vi "Update Connect Panel Doc.vi"(8 "error in (no error)":errorcluster, 11 "vi path":path) -> (0 "error out":errorcluster, 3 "Array":T1(array[cluster]))   [LabVIEW 2017]
uses:
  Communicable State Machine.lvlib
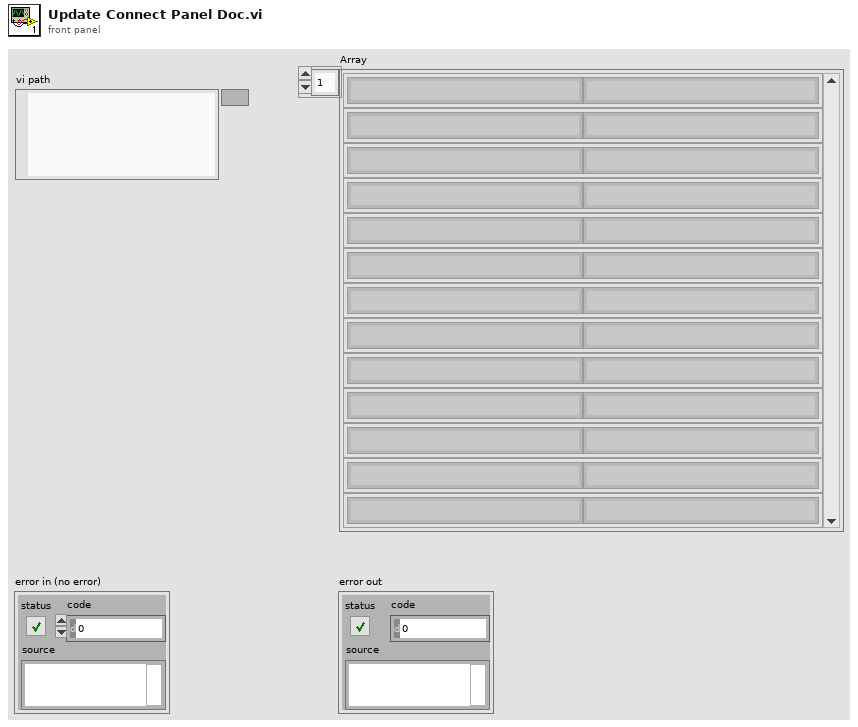
[diagram p1: front panel]
types:
  T1 = cluster{"Label.Text":string, "Label.Text":string}[]
  T2 = cluster{"Label.Text":string, "delimited string":string}
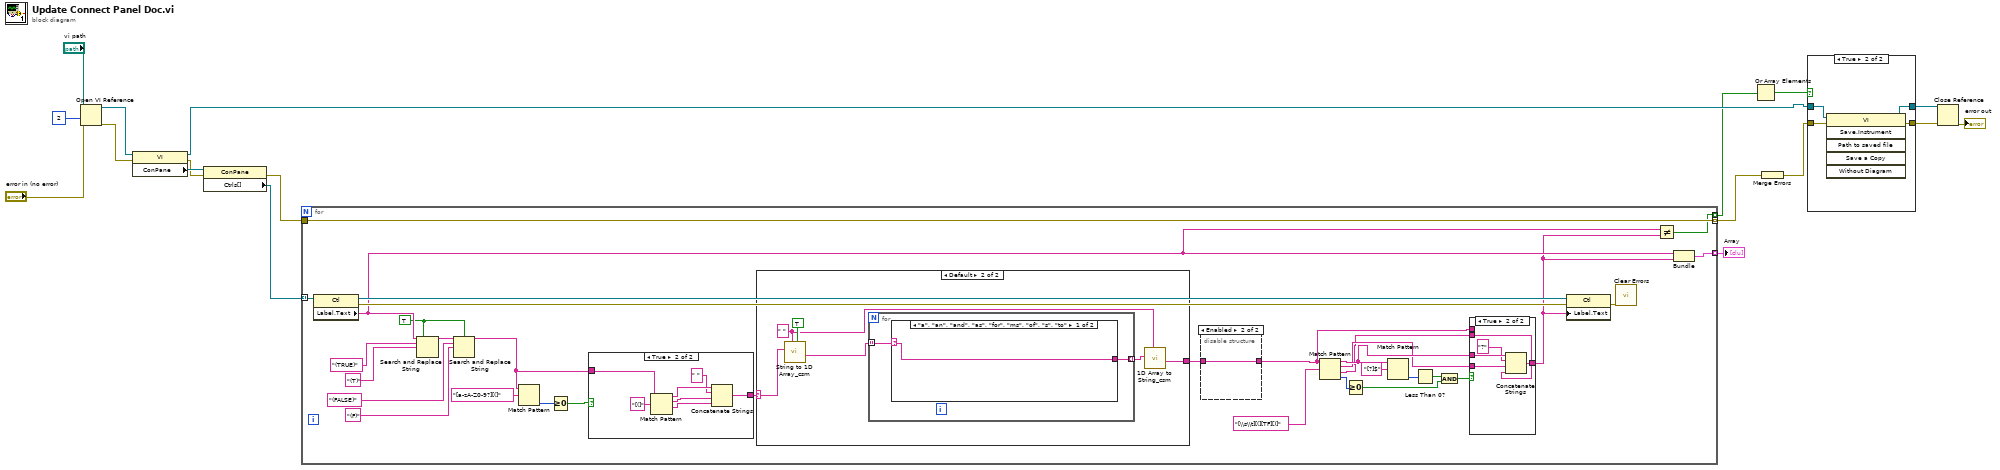
[diagram p0: block diagram]
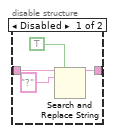
[diagram p4: hidden frame]
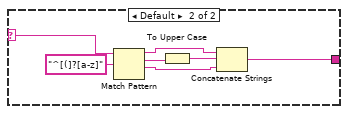
[diagram p6: hidden frame]
diagram:
  n1 = Open VI Reference(vi path="vi path", options=2, error in (no error)="error in (no error)") -> (vi reference=w17:refnum<vi>, error out=w14:errorcluster)  [unwired: 3 in]
  n2 = property class="VI"(reference=w17, error in=w14) -> (reference out=w9:refnum<vi>, error out=w15:errorcluster, "ConPane"=w16:refnum<vi>)
  n3 = property class="ConPane"(reference=w16, error in=w15) -> (error out=w11:errorcluster, "Ctrls[]"=w12:refnum<vi>[])  [unwired: 1 out]
  n4 = for {
    tunnel: w12 -> [w50] mode=indexing
    tunnel: [w44] -> w1 mode=indexing
    tunnel: [w49] -> w10 mode=indexing
    tunnel: w11 -> [w49]
    tunnel: [w40] -> w5 mode=indexing
    w35 = TRUE ("replace all? (F)")
    n5 = property class="Ctl"(reference=w50) -> (reference out=w47:refnum<vi>, error out=w46:errorcluster, "Label.Text"=w38:string)  [unwired: 1 in]
    n6 = Search and Replace String(replace all?=w35, input string=w38, search string="(TRUE)" ("Label.Text"), replace string="(T)" ("Label.Text")) -> (result string=w37:string)  [unwired: 4 in, 3 out]
    n7 = Search and Replace String(case sensitive?=w35, input string=w37, search string="(FALSE)" ("Label.Text"), replace string="(F)" ("Label.Text")) -> (result string=w36:string)  [unwired: 4 in, 3 out]
    n8 = Match Pattern(string=w36, regular expression="[a-zA-Z0-9?][(]") -> (offset past match=w45:i32)  [unwired: 1 in, 3 out]
    n9 = Greater Or Equal To 0?(x=w45) -> (x >= 0?=w42:bool)
    n10 = case shown="True" w42 {
      tunnel: w36 -> [w79 w86]
      tunnel: [w79 w85] -> w41
      frame False {
      }
      frame True {
        n11 = Match Pattern(string=w86, regular expression="[(]") -> (before substring=w83:string, match substring=w81:string, after substring=w82:string)  [unwired: 1 in, 1 out]
        n12 = Concatenate Strings(w83, " " ("regular expression"), w81, w82) -> (w85:string)
      }
    }
    n13 = case shown="Default" w41 {
      selector: w41 -> [w62 w68]
      tunnel: [w62 w63] -> w39
      frame "error in (no error)", "error out" {
      }
      frame Default {
        w64 = " " ("delimiter (Tab)")
        n14 = call "String to 1D Array_csm.vi"("ignore duplicate delimiters? (F=No)"=TRUE, "delimiter (Tab)"=w64, "string"=w68) -> ("Array of Strings"=w66:string[])  [unwired: 8 in]
        n15 = for {
          tunnel: w66 -> [w70] mode=indexing
          tunnel: [w69] -> w65 mode=indexing
          n16 = case shown="\"a\", \"an\", \"and\", \"as\", \"for\", \"ms\", \"of\", \"s\", \"to\"" w70 {
            selector: w70 -> [w71 w78]
            tunnel: [w71 w72] -> w69
            frame "a", "an", "and", "as", "for", "ms", "of", "s", "to" {
            }
            frame Default {
              n17 = Match Pattern(string=w78, regular expression="^[(]?[a-z]") -> (before substring=w74:string, match substring=w76:string, after substring=w73:string)  [unwired: 1 in, 1 out]
              n18 = To Upper Case(1:w76) -> (0:w75:string)
              n19 = Concatenate Strings(w74, w75, w73) -> (w72:string)
            }
          }
        }
        n20 = call "1D Array to String_csm.vi"("delimiter (Tab)"=w64, "Array of Strings"=w65) -> ("delimited string"=w63:string)  [unwired: 9 in]
      }
    }
    n21 = disable-structure shown="Enabled" {
      disable-tunnel: [w60 w61] -> w19
      disable-tunnel: w39 -> [w59 w61]
      frame Disabled {
        n22 = Search and Replace String(replace all?=TRUE ("replace all? (F)"), input string=w59, search string="?" ("regular expression")) -> (result string=w60:string)  [unwired: 5 in, 3 out]
      }
      frame Enabled {
      }
    }
    n23 = Match Pattern(string=w19, regular expression="[\\s\\t][(][TF][)]") -> (before substring=w23:string, match substring=w22:string, after substring=w21:string, offset past match=w29:i32)  [unwired: 1 in]
    n24 = Greater Or Equal To 0?(x=w29) -> (x >= 0?=w25:bool)
    n25 = Match Pattern(string=w23, regular expression="[?]$") -> (offset past match=w27:i32)  [unwired: 1 in, 3 out]
    n26 = Less Than 0?(x=w27) -> (x < 0?=w26:bool)
    n27 = And(x=w26, y=w25) -> (x .and. y?=w24:bool)
    n28 = case shown="True" w24 {
      tunnel: w23 -> [_ w56]
      tunnel: w22 -> [_ w54]
      tunnel: w21 -> [_ w53]
      tunnel: [w51 w52] -> w20
      tunnel: w19 -> [w51 _]
      frame False {
      }
      frame True {
        n29 = Concatenate Strings(w56, "?" ("regular expression"), w54, w53) -> (w52:string)
      }
    }
    n30 = property class="Ctl"(reference=w47, error in=w46, "Label.Text"=w20) -> (error out=w43:errorcluster)  [unwired: 1 out]
    n31 = call <vilib>:"Clear Errors.vi"("error in (no error)"=w43) -> ()  [unwired: 5 in, 2 out]
    n32 = Not Equal?(x=w38, y=w20) -> (x != y?=w40:bool)
    n33 = Bundle("Label.Text"=w38, "delimited string"=w20) -> (w44:T2)  [unwired: 1 in]
  }
  "Array" <- w1
  n34 = Or Array Elements(Boolean array=w5) -> (logical OR=w4:bool)
  n35 = Merge Errors(w10) -> (w6:errorcluster)
  n36 = case shown="True" w4 {
    tunnel: [w88 w92] -> w7
    tunnel: [w87 w91] -> w8
    tunnel: w6 -> [w88 w89]
    tunnel: w9 -> [w87 w90]
    frame False {
    }
    frame True {
      n37 = invoke class="VI" method="Save.Instrument"(reference=w90, error in=w89) -> (reference out=w91:refnum<vi>, error out=w92:errorcluster)  [unwired: 4 in, 4 out]
    }
  }
  n38 = Close Reference(reference=w8, error in (no error)=w7) -> (error out=→"error out":errorcluster)
